vi "checkout.vi"(7 "locked by?":string, 8 "error in (no error)":errorcluster) -> (0 "error out":errorcluster, 3 "GeneralAnalyser out":refnum<class "GenericAnalyser.lvclass">)   [LabVIEW 2010, in "GenericAnalyser.lvclass"]
uses:
  GenericAnalyser.lvclass
  class_data.vi
  common/classes/ErrorController/ErrorController/class_data.vi
  common/classes/GenericComponent/GenericComponent/GenericComponent.lvclass
  common/classes/ErrorController/ErrorController/ErrorController.lvclass
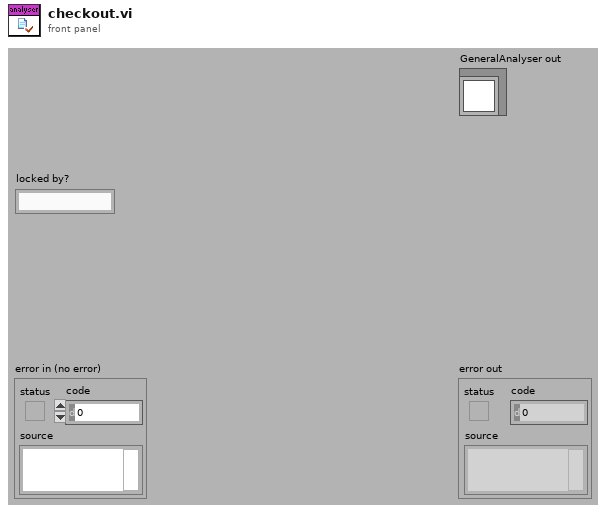
[diagram p1: front panel]
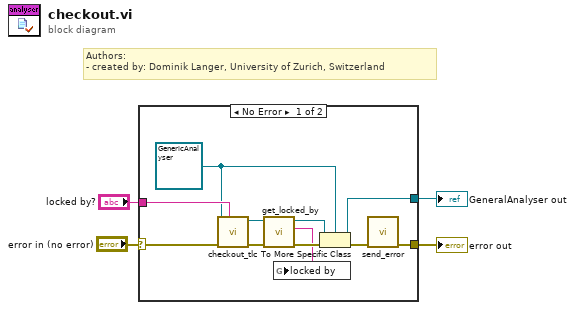
[diagram p0: block diagram]
diagram:
  # "Authors: \n- created by: Dominik Langer, University of Zurich, Switzerland"
  n1 = case shown="No Error" "error in (no error)" {
    selector: "error in (no error)" -> [w9 w16]
    tunnel: [w6 w16] -> w3
    tunnel: [w10 _] -> w2
    tunnel: "locked by?" -> [w8 _]
    frame No Error {
      w5 = refnum<class "GenericAnalyser.lvclass"> refnum ("GeneralAnalyser.lvclass")
      n2 = call-dynamic "checkout_tlc.vi"("locked by?"=w8, "error in (no error)"=w9, "GenericToplevelComponent in"=w5) -> ("error out"=w15:errorcluster, "GenericToplevelComponent out"=w14:refnum<class "GenericToplevelComponent.lvclass">)  [unwired: 7 in]
      n3 = call "get_locked_by.vi"("error in (no error)"=w15, "GenericPlugin.lvclass in"=w14) -> ("error out"=w13:errorcluster, "locked by"=w11:string, "GenericPlugin.lvclass out"=w12:refnum<class "GenericToplevelComponent.lvclass">)  [unwired: 7 out]
      n4 = global write "class_data.vi" "locked by"(w11) -> ()
      n5 = To More Specific Class(target class=w5, reference=w12, error in=w13) -> (specific class reference=w10:refnum<class "GenericAnalyser.lvclass">, error out=w7:errorcluster)
      n6 = call "send_error.vi"("error in (no error)"=w7) -> ("error out"=w6:errorcluster)  [unwired: 10 in]
    }
    frame Error {
    }
  }
  "error out" <- w3
  "GeneralAnalyser out" <- w2
